vi "MathCad_Matrix_Get_Elmnt.vi"(4 "row":i32, 6 "col":i32, 7 "error in":errorcluster, 8 "Mathcad.IMatrixValue Refnum":refnum<k7>) -> (0 "error out":errorcluster, 1 "GetElement":variant, 2 "Mathcad.IMatrixValue Refnum":refnum<k7>)   [LabVIEW 2015]
doc: "Gets the value from the reference retrieved from the getrefnum VI."
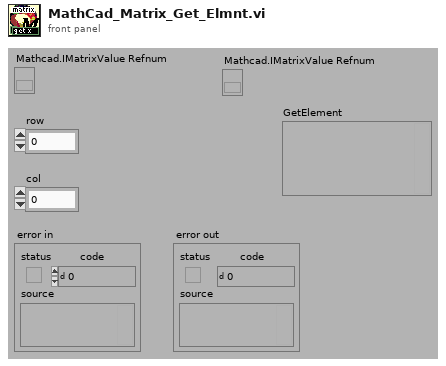
[diagram p1: front panel]
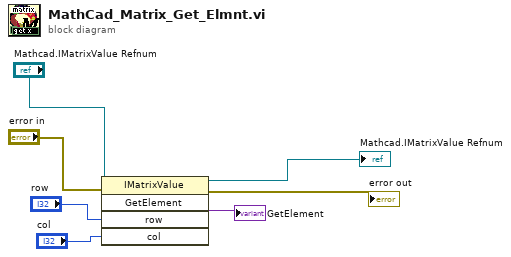
[diagram p0: block diagram]
diagram:
  n1 = invoke class="IMatrixValue" method="GetElement"(reference="Mathcad.IMatrixValue Refnum", error in="error in", "row"="row", "col"="col") -> (reference out=→"Mathcad.IMatrixValue Refnum":refnum<k7>, error out=→"error out":errorcluster, "GetElement"=→"GetElement":variant)  [unwired: 1 in, 2 out]
